vi "dfd_TF to Filter Coef.vi"(7 "type":T2=enum."IIR Direct Form II Transposed", 8 "error in (no error)":errorcluster, 10 "denominator":dbl[](array[numeric])=[1.0] format="%.2f", 11 "numerator":dbl[](array[numeric])=[1.0] format="%.2f") -> (0 "error out":errorcluster, 3 "filter coef":T1)   [LabVIEW 2017, in "NI_DigFilterLicensed.lvlib"]
uses:
  <vilib>/addons/Digital Filter Design/NI_DigFilterLicensed.lvlib
  <vilib>/addons/Digital Filter Design/_Objects.llb/DFD Filter Structure Type Selector.ctl
  <vilib>/addons/Digital Filter Design/_Objects.llb/DFD Filter Coef.ctl
  <vilib>/addons/Digital Filter Design/_Misc.llb/dfd_Error Handlers (Single).vi
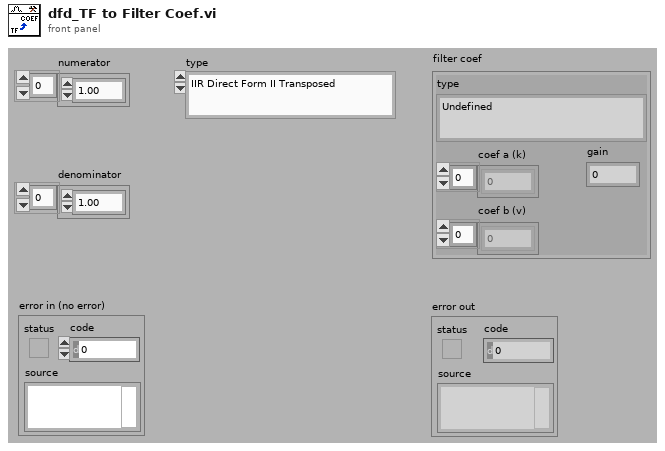
[diagram p1: front panel]
types:
  T1 = typedef "NI_DigFilterLicensed.lvlib/DFD Filter Coef.ctl" = cluster{"type":T2, "gain":dbl, "coef a (k)":dbl[], "coef b (v)":dbl[]}
  T2 = typedef "NI_DigFilterLicensed.lvlib/DFD Filter Structure Type Selector.ctl" = enum16{"Undefined", "FIR Direct Form", "FIR Direct Form Transposed", "FIR Symmetric", "FIR Antisymmetric", "IIR Direct Form I", "IIR Direct Form I Transposed", "IIR Direct Form II", "IIR Direct Form II Transposed", "IIR Cascaded Second Order Sections Form I", "IIR Cascaded Second Order Sections Form I Transposed", "IIR Cascaded Second Order Sections Form II", "IIR Cascaded Second Order Sections Form II Transposed", "Lattice Allpass (basic sections)", "Lattice Allpass (one multiplier sections)", "Lattice Allpass (normalized sections)", "Lattice AR (basic sections)", "Lattice AR (one multiplier sections)", "Lattice AR (normalized sections)", "Lattice MA (minimum phase)", "Lattice MA (maximum phase)", "Lattice ARMA (basic sections)", "Lattice ARMA (one multiplier sections)", "Lattice ARMA (normalized sections)"}
  T3 = enum16{"Basic Section", "One Multiplier Section", "Normalized Section"}
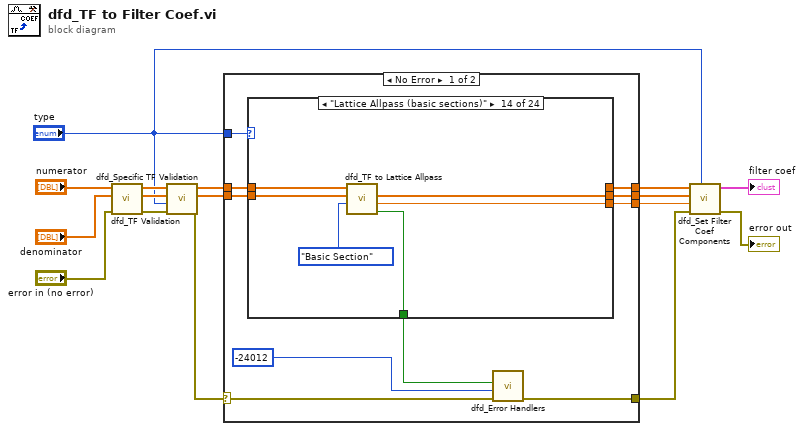
[diagram p0: block diagram]
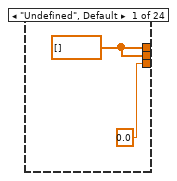
[diagram p2: hidden frame]
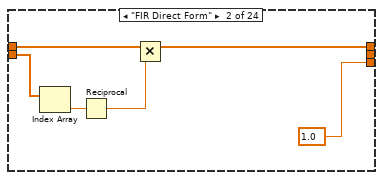
[diagram p3: hidden frame]
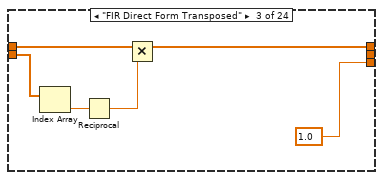
[diagram p4: hidden frame]
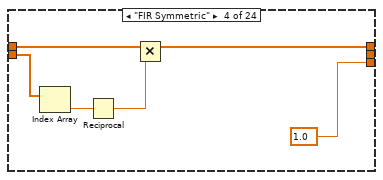
[diagram p5: hidden frame]
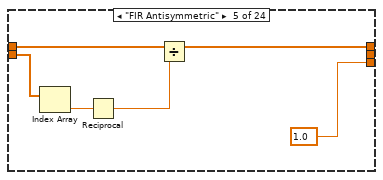
[diagram p6: hidden frame]
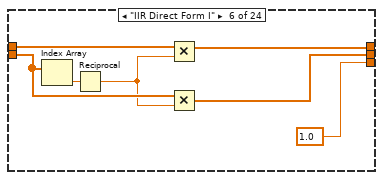
[diagram p7: hidden frame]
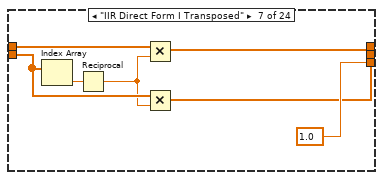
[diagram p8: hidden frame]
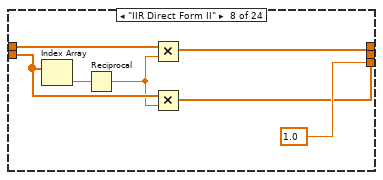
[diagram p9: hidden frame]
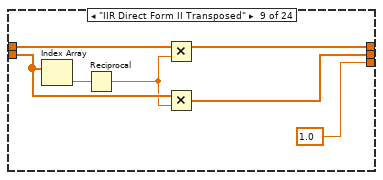
[diagram p10: hidden frame]
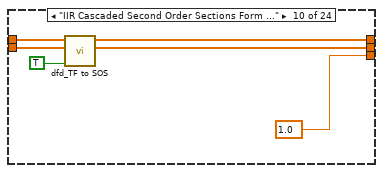
[diagram p11: hidden frame]
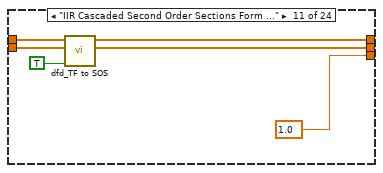
[diagram p12: hidden frame]
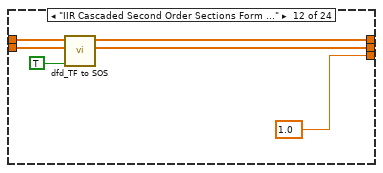
[diagram p13: hidden frame]
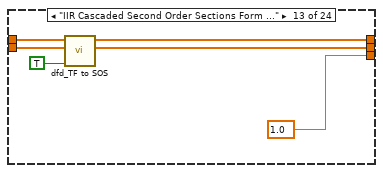
[diagram p14: hidden frame]
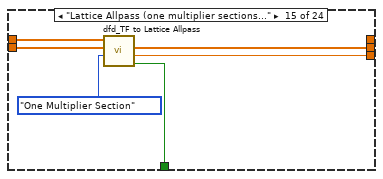
[diagram p15: hidden frame]
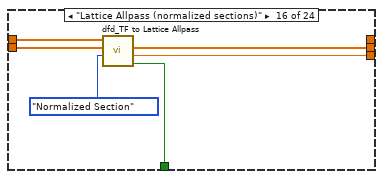
[diagram p16: hidden frame]
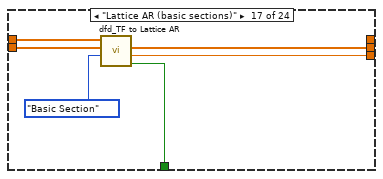
[diagram p17: hidden frame]
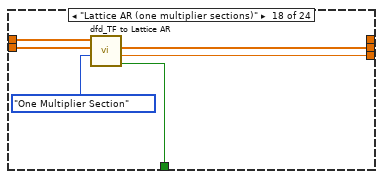
[diagram p18: hidden frame]
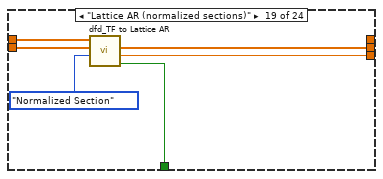
[diagram p19: hidden frame]
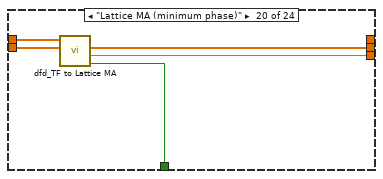
[diagram p20: hidden frame]
diagram:
  n1 = call <vilib>:"dfd_TF Validation.vi"("error in (no error)"="error in (no error)", "denominator"="denominator", "numerator"="numerator") -> ("error out"=w5:errorcluster, "validated denominator"=w7:dbl[], "validated numerator"=w8:dbl[])  [unwired: 3 out]
  n2 = call <vilib>:"dfd_Specific TF Validation.vi"("error in (no error)"=w5, "type"="type", "denominator"=w7, "numerator"=w8) -> ("error out"=w3:errorcluster, "dup denominator"=w1:dbl[], "dup numerator"=w2:dbl[])  [unwired: 5 out]
  n3 = case shown="No Error" w3 {
    selector: w3 -> [w20 w173]
    tunnel: w2 -> [w26 _]
    tunnel: w1 -> [w25 _]
    tunnel: [w24 _] -> w16
    tunnel: [w23 _] -> w15
    tunnel: [w22 _] -> w14
    tunnel: [w19 w173] -> w13
    tunnel: "type" -> [w21 _]
    frame No Error {
      n4 = case shown="\"Lattice Allpass (basic sections)\"" w21 {
        tunnel: w26 -> [_ w32 w38 w44 w50 w59 w66 w73 w80 w86 w92 w98 w104 w110 w116 w122 w125 w131 w138 w145 w151 w157 w165 w172]
        tunnel: w25 -> [_ w33 w39 w45 w51 w58 w65 w72 w79 w85 w91 w97 w103 w109 w115 w121 w128 w134 w140 w143 w148 w156 w164 w171]
        tunnel: [w28 w31 w36 w42 w48 w54 w61 w68 w75 w84 w90 w96 w102 _ _ _ _ _ _ _ _ w155 w161 w168] -> w24
        tunnel: [w28 _ _ _ _ w55 w62 w69 w76 w83 w89 w95 w101 w106 w112 w118 w126 w132 w136 w141 w146 w158 w159 w166] -> w23
        tunnel: [0.0 ("gain") 1.0 ("gain") 1.0 ("gain") 1.0 ("gain") 1.0 ("gain") 1.0 ("gain") 1.0 ("gain") 1.0 ("gain") 1.0 ("gain") 1.0 ("gain") 1.0 ("gain") 1.0 ("gain") 1.0 ("gain") w107 w113 w119 w124 w130 w137 w142 w147 1.0 ("gain") 1.0 ("gain") 1.0 ("gain")] -> w22
        tunnel: [_ _ _ _ _ _ _ _ _ _ _ _ _ w108 w114 w120 w127 w133 w139 w144 w149 w153 w162 w169] -> w18
        frame "Undefined", Default {
          w28 = dbl[] [] ("v")
        }
        frame "FIR Direct Form" {
          n5 = Index Array(array=w33) -> (element=w30:dbl)  [unwired: 1 in]
          n6 = Reciprocal(x=w30) -> (1/x=w29:dbl)
          n7 = Multiply(x=w32, y=w29) -> (x*y=w31:dbl[])
        }
        frame "FIR Direct Form Transposed" {
          n8 = Index Array(array=w39) -> (element=w37:dbl)  [unwired: 1 in]
          n9 = Reciprocal(x=w37) -> (1/x=w35:dbl)
          n10 = Multiply(x=w38, y=w35) -> (x*y=w36:dbl[])
        }
        frame "FIR Symmetric" {
          n11 = Index Array(array=w45) -> (element=w43:dbl)  [unwired: 1 in]
          n12 = Reciprocal(x=w43) -> (1/x=w41:dbl)
          n13 = Multiply(x=w44, y=w41) -> (x*y=w42:dbl[])
        }
        frame "FIR Antisymmetric" {
          n14 = Index Array(array=w51) -> (element=w49:dbl)  [unwired: 1 in]
          n15 = Reciprocal(x=w49) -> (1/x=w47:dbl)
          n16 = Divide(x=w50, y=w47) -> (x/y=w48:dbl[])
        }
        frame "IIR Direct Form I" {
          n17 = Index Array(array=w58) -> (element=w57:dbl)  [unwired: 1 in]
          n18 = Reciprocal(x=w57) -> (1/x=w53:dbl)
          n19 = Multiply(x=w59, y=w53) -> (x*y=w54:dbl[])
          n20 = Multiply(x=w58, y=w53) -> (x*y=w55:dbl[])
        }
        frame "IIR Direct Form I Transposed" {
          n21 = Index Array(array=w65) -> (element=w64:dbl)  [unwired: 1 in]
          n22 = Reciprocal(x=w64) -> (1/x=w60:dbl)
          n23 = Multiply(x=w66, y=w60) -> (x*y=w61:dbl[])
          n24 = Multiply(x=w65, y=w60) -> (x*y=w62:dbl[])
        }
        frame "IIR Direct Form II" {
          n25 = Index Array(array=w72) -> (element=w71:dbl)  [unwired: 1 in]
          n26 = Reciprocal(x=w71) -> (1/x=w67:dbl)
          n27 = Multiply(x=w73, y=w67) -> (x*y=w68:dbl[])
          n28 = Multiply(x=w72, y=w67) -> (x*y=w69:dbl[])
        }
        frame "IIR Direct Form II Transposed" {
          n29 = Index Array(array=w79) -> (element=w78:dbl)  [unwired: 1 in]
          n30 = Reciprocal(x=w78) -> (1/x=w74:dbl)
          n31 = Multiply(x=w80, y=w74) -> (x*y=w75:dbl[])
          n32 = Multiply(x=w79, y=w74) -> (x*y=w76:dbl[])
        }
        frame "IIR Cascaded Second Order Sections Form I" {
          n33 = call <vilib>:"dfd_TF to SOS.vi"("UP?"=TRUE, "denominator"=w85, "numerator"=w86) -> ("SOS reverse coefficients"=w83:dbl[], "SOS forward coefficients"=w84:dbl[])  [unwired: 7 out]
        }
        frame "IIR Cascaded Second Order Sections Form I Transposed" {
          n34 = call <vilib>:"dfd_TF to SOS.vi"("UP?"=TRUE, "denominator"=w91, "numerator"=w92) -> ("SOS reverse coefficients"=w89:dbl[], "SOS forward coefficients"=w90:dbl[])  [unwired: 7 out]
        }
        frame "IIR Cascaded Second Order Sections Form II" {
          n35 = call <vilib>:"dfd_TF to SOS.vi"("UP?"=TRUE, "denominator"=w97, "numerator"=w98) -> ("SOS reverse coefficients"=w95:dbl[], "SOS forward coefficients"=w96:dbl[])  [unwired: 7 out]
        }
        frame "IIR Cascaded Second Order Sections Form II Transposed" {
          n36 = call <vilib>:"dfd_TF to SOS.vi"("UP?"=TRUE, "denominator"=w103, "numerator"=w104) -> ("SOS reverse coefficients"=w101:dbl[], "SOS forward coefficients"=w102:dbl[])  [unwired: 7 out]
        }
        frame "Lattice Allpass (basic sections)" {
          n37 = call <vilib>:"dfd_TF to Lattice Allpass.vi"("section type"=T3."Basic Section", "denominator"=w109, "numerator"=w110) -> ("failed?"=w108:bool, "gain"=w107:dbl, "k [1~M]"=w106:dbl[])  [unwired: 6 out]
        }
        frame "Lattice Allpass (one multiplier sections)" {
          n38 = call <vilib>:"dfd_TF to Lattice Allpass.vi"("section type"=T3."One Multiplier Section", "denominator"=w115, "numerator"=w116) -> ("failed?"=w114:bool, "gain"=w113:dbl, "k [1~M]"=w112:dbl[])  [unwired: 6 out]
        }
        frame "Lattice Allpass (normalized sections)" {
          n39 = call <vilib>:"dfd_TF to Lattice Allpass.vi"("section type"=T3."Normalized Section", "denominator"=w121, "numerator"=w122) -> ("failed?"=w120:bool, "gain"=w119:dbl, "k [1~M]"=w118:dbl[])  [unwired: 6 out]
        }
        frame "Lattice AR (basic sections)" {
          n40 = call <vilib>:"dfd_TF to Lattice AR.vi"("section type"=T3."Basic Section", "denominator"=w128, "numerator"=w125) -> ("fail?"=w127:bool, "gain"=w124:dbl, "k [1~M]"=w126:dbl[])  [unwired: 6 out]
        }
        frame "Lattice AR (one multiplier sections)" {
          n41 = call <vilib>:"dfd_TF to Lattice AR.vi"("section type"=T3."One Multiplier Section", "denominator"=w134, "numerator"=w131) -> ("fail?"=w133:bool, "gain"=w130:dbl, "k [1~M]"=w132:dbl[])  [unwired: 6 out]
        }
        frame "Lattice AR (normalized sections)" {
          n42 = call <vilib>:"dfd_TF to Lattice AR.vi"("section type"=T3."Normalized Section", "denominator"=w140, "numerator"=w138) -> ("fail?"=w139:bool, "gain"=w137:dbl, "k [1~M]"=w136:dbl[])  [unwired: 6 out]
        }
        frame "Lattice MA (minimum phase)" {
          n43 = call <vilib>:"dfd_TF to Lattice MA.vi"("denominator"=w143, "numerator"=w145) -> ("fail?"=w144:bool, "gain"=w142:dbl, "k [1~M]"=w141:dbl[])  [unwired: 7 out]
        }
        frame "Lattice MA (maximum phase)" {
          n44 = Reverse 1D Array(array=w151) -> (reversed array=w150:dbl[])
          n45 = call <vilib>:"dfd_TF to Lattice MA.vi"("denominator"=w148, "numerator"=w150) -> ("fail?"=w149:bool, "gain"=w147:dbl, "k [1~M]"=w146:dbl[])  [unwired: 7 out]
        }
        frame "Lattice ARMA (basic sections)" {
          n46 = call <vilib>:"dfd_TF to Lattice ARMA.vi"("section type"=T3."Basic Section", "denominator"=w156, "numerator"=w157) -> ("fail?"=w153:bool, "k [1~M]"=w158:dbl[], "v [0~M]"=w155:dbl[])  [unwired: 6 out]
        }
        frame "Lattice ARMA (one multiplier sections)" {
          n47 = call <vilib>:"dfd_TF to Lattice ARMA.vi"("section type"=T3."One Multiplier Section", "denominator"=w164, "numerator"=w165) -> ("fail?"=w162:bool, "k [1~M]"=w159:dbl[], "v [0~M]"=w161:dbl[])  [unwired: 6 out]
        }
        frame "Lattice ARMA (normalized sections)" {
          n48 = call <vilib>:"dfd_TF to Lattice ARMA.vi"("section type"=T3."Normalized Section", "denominator"=w171, "numerator"=w172) -> ("fail?"=w169:bool, "k [1~M]"=w166:dbl[], "v [0~M]"=w168:dbl[])  [unwired: 6 out]
        }
      }
      n49 = call-poly <vilib>:"dfd_Error Handlers.vi"("error in (no error)"=w20, "error code"=-24012 ("ERR_INCOMPATIBLE_STRUT"), "condition failed?"=w18) -> ("error out"=w19:errorcluster)  [unwired: 8 out]
    }
    frame Error {
    }
  }
  n50 = call <vilib>:"dfd_Set Filter Coef Components.vi"("type"="type", "error in (no error)"=w13, "gain"=w14, "coef a (k)"=w15, "coef b (v)"=w16) -> ("error out"=→"error out":errorcluster, "filter coef"=→"filter coef":T1)  [unwired: 5 out]
